vi "KINECT_Calibrate.vi"(6 "Arm Drive Min in (Reverse)":dbl, 7 "Enable Calibration":bool, 8 "Current Value":dbl, 9 "Wait Time (ms)":u32=5000, 10 "Arm Drive Max in (Forward)":dbl) -> (0 "Arm Drive Min out (Reverse)":dbl, 1 "Arm Drive Max out (Forward)":dbl, 2 "Calibrating":bool, 3 "Result":T1(ring))   [LabVIEW 2011]
panel:
  in  "Value 1":dbl
  in  "Old Time":u32
  in  "Baseline":dbl
  in  "Repeated":bool
  in  "Enum":T1(ring)
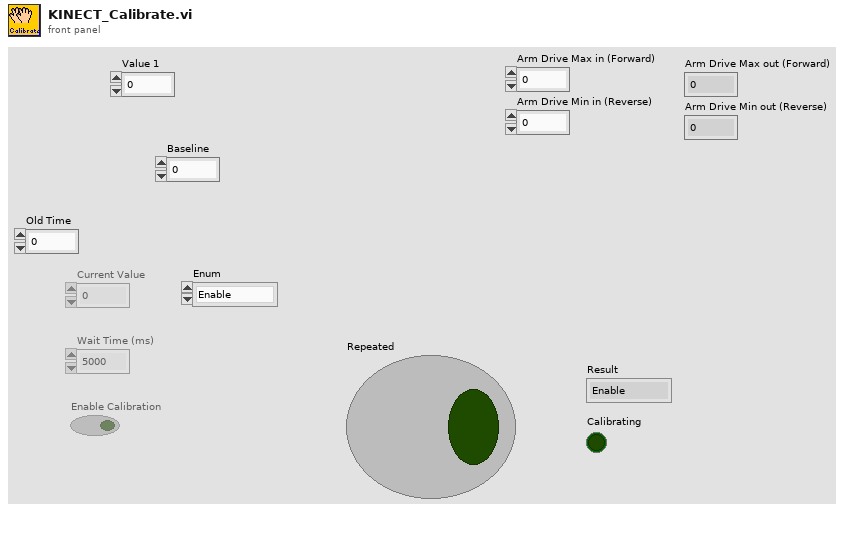
[diagram p1: front panel]
types:
  T1 = enum16{"Enable", "Set/Reset", "Run Timer", "Read/Store"}
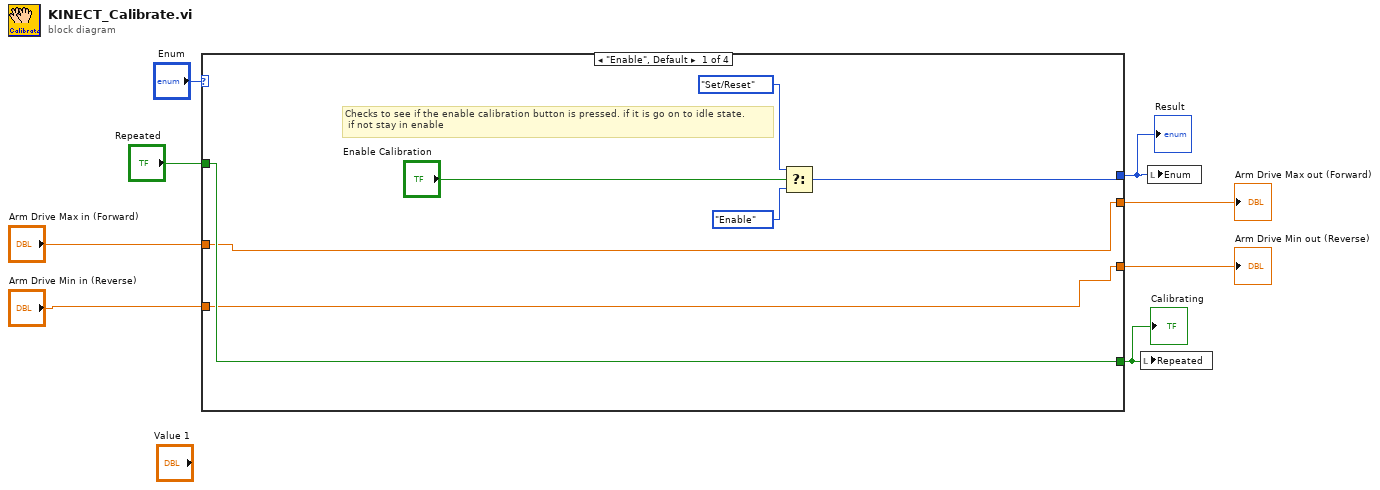
[diagram p0: block diagram]
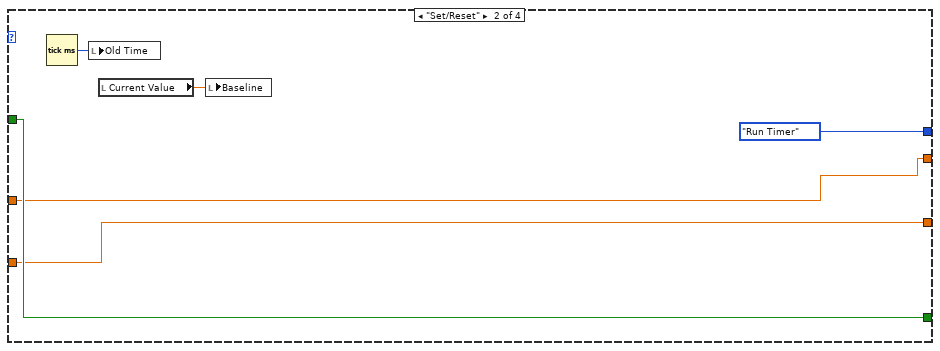
[diagram p2: hidden frame]
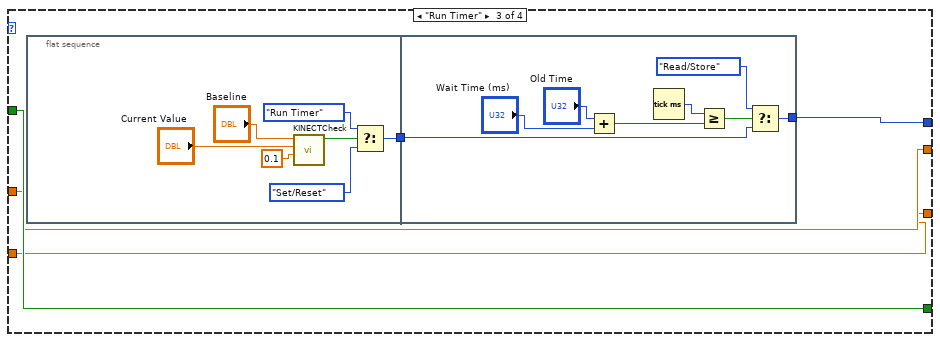
[diagram p3: hidden frame]
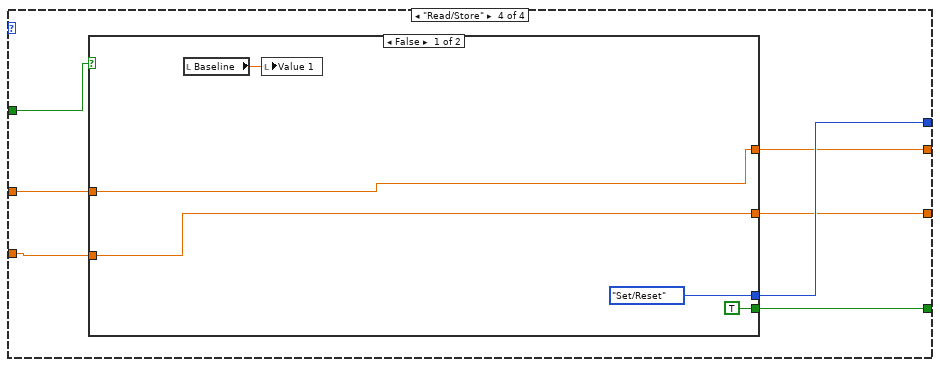
[diagram p4: hidden frame]
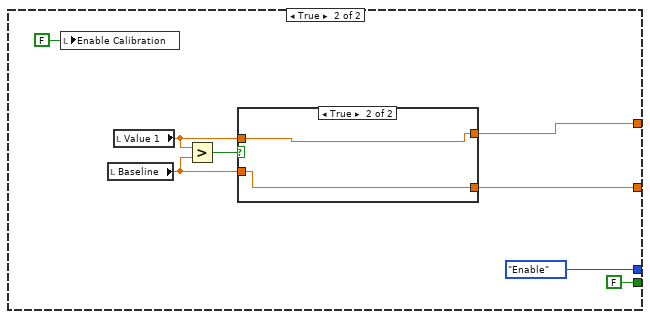
[diagram p5: hidden frame]
diagram:
  n1 = case shown="\"Enable\", Default" "Enum" {
    tunnel: [w12 T1."Run Timer" ("Enum") w25 w48] -> w6
    tunnel: [w11 w18 w24 w47] -> w5
    tunnel: "Repeated" -> [w11 w18 w24 w46]
    tunnel: [w10 w17 w23 w45] -> w4
    tunnel: [w9 w16 w22 w44] -> w3
    tunnel: "Arm Drive Max in (Forward)" -> [w10 w17 w23 w43]
    tunnel: "Arm Drive Min in (Reverse)" -> [w9 w16 w22 w42]
    frame "Enable", Default {
      # "Checks to see if the enable calibration button is pressed. if it is go on to idle state.\n if not stay in enable"
      n2 = Select(t=T1."Set/Reset" ("Enum"), s="Enable Calibration", f=T1."Enable" ("Enum")) -> (s? t:f=w12:T1)
    }
    frame "Set/Reset" {
      n3 = Tick Count (ms)() -> (millisecond timer value=w21:u32)
      n4 = local write "Old Time"(w21) -> ()
      n5 = local read "Current Value"() -> (w20:dbl)
      n6 = local write "Baseline"(w20) -> ()
    }
    frame "Run Timer" {
      n7 = flat-sequence {
        tunnel: [w33] -> w26
        tunnel: w26 -> [w41]
        tunnel: [w40] -> w25
        frame #0 {
          n8 = call "KINECTCheck.vi"("Delta"=0.1, "Current"="Current Value", "Baseline"="Baseline") -> ("In Range?"=w27:bool)  [unwired: 8 in]
          n9 = Select(t=T1."Run Timer" ("Enum"), s=w27, f=T1."Set/Reset" ("Enum")) -> (s? t:f=w33:T1)
        }
        frame #1 {
          n10 = Add(x="Old Time", y="Wait Time (ms)") -> (x+y=w38:u32)
          n11 = Tick Count (ms)() -> (millisecond timer value=w37:u32)
          n12 = Greater Or Equal?(x=w37, y=w38) -> (x >= y?=w34:bool)
          n13 = Select(t=T1."Read/Store" ("Enum"), s=w34, f=w41) -> (s? t:f=w40:T1)
        }
      }
    }
    frame "Read/Store" {
      n14 = case shown="False" w46 {
        tunnel: [T1."Set/Reset" ("Enum") T1."Enable" ("Enum")] -> w48
        tunnel: [TRUE FALSE] -> w47
        tunnel: [w50 w55] -> w45
        tunnel: [w49 w54] -> w44
        tunnel: w43 -> [w50 _]
        tunnel: w42 -> [w49 _]
        frame False {
          n15 = local read "Baseline"() -> (w51:dbl)
          n16 = local write "Value 1"(w51) -> ()
        }
        frame True {
          n17 = local write "Enable Calibration"(FALSE ("Enable Calibration")) -> ()
          n18 = local read "Baseline"() -> (w56:dbl)
          n19 = local read "Value 1"() -> (w57:dbl)
          n20 = Greater?(x=w57, y=w56) -> (0:w58:bool)
          n21 = case shown="True" w58 {
            tunnel: w57 -> [w62 w65]
            tunnel: w56 -> [w63 w64]
            tunnel: [w63 w65] -> w55
            tunnel: [w62 w64] -> w54
            frame False {
            }
            frame True {
            }
          }
        }
      }
    }
  }
  "Result" <- w6
  "Calibrating" <- w5
  "Arm Drive Max out (Forward)" <- w4
  "Arm Drive Min out (Reverse)" <- w3
  n22 = local write "Repeated"(w5) -> ()
  n23 = local write "Enum"(w6) -> ()
